vi "float_to_real_5x3.vi"(10 "Float":dbl) -> (2 "REAL_5X3":string)   [LabVIEW 2018, in "Inficon IC6.lvlib"]
doc: "Format a float as an IC6 defined REAL_5X3 string."
uses:
  <instrlib>/Inficon IC6/Inficon IC6.lvlib
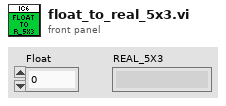
[diagram p1: front panel]
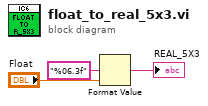
[diagram p0: block diagram]
diagram:
  n1 = Format Value(format string="%06.3f", value (0)="Float") -> (output string=→"REAL_5X3":string)  [unwired: 1 in]
